vi "Dashboard Main.vi"() -> ()   [LabVIEW 2016]
uses:
  <vilib>/Utility/miscctls.llb/LVRowAndColumnTypeDef.ctl
  <vilib>/event_ctls.llb/eventvkey.ctl
  <vilib>/Rock Robotics/Network Tables/NT Read Boolean.vi
  <vilib>/Rock Robotics/WPI/Dashboard/WPI_DashboardLogging Global.vi
panel:
  in  "Camera Settings Right":T1={"Frame Rate"=30, "Compression"=30, "Size"=1, "DB Camera Config"=FALSE} {"Frame Rate" scale=1.0..30.0; "Compression" scale=100.0..-1.0; "Size" items=["640x480", "320x240", "160x120"]}
  in  "Camera Name Right":string(combo)="No Camera Selection"
  out "Camera Info":cluster{"Mbps LED":bool, "Mbps":dbl, "fps":dbl} {"fps" format="%#.1g"; "Mbps" format="%#.1g"}
  in  "Camera Settings":T1={"Frame Rate"=30, "Compression"=30, "Size"=1, "DB Camera Config"=FALSE} {"Frame Rate" scale=1.0..30.0; "Compression" scale=100.0..-1.0; "Size" items=["640x480", "320x240", "160x120"]}
  in  "TCP":refnum<k5>
  in  "Rec Mode":enum32{"Stop", "Record", "Playback"}(radio)
  out "Robot IP":string
  out "Image Message":string="Timeout in Camera Communications"
  in  "Dashboard Tab":T2(tab)
  out "?":string="CHOOSE AN AUTONOMOUS MODE!!!"
  in  "Select Auto":string(combo)="Select Autonomous ..."
  out "NT Connection":bool
  out "JS1 Z":dbl(slide) scale=-1.0..1.0 scale format="%#_2e"
  out "JS1 Graph":cluster{"X":dbl, "Y":dbl}[](graph)
  out "JS1 Buttons":T3
  out "JS2 Z":dbl(slide) scale=-1.0..1.0 scale format="%#_2e"
  out "JS2 Graph":cluster{"X":dbl, "Y":dbl}[](graph)
  out "JS2 Buttons":T3
  out "Mode":T4(ring)=enum."Auto Disabled"
  out "Camera Image Right":T5(plugin-control)
  out "Mid":dbl(slide) scale=0.0..320.0
  out "Targets Found?":bool
  out "?":string="Cortechs Robotics\nSteamworks 2017"
  out "Low Gear?":bool
  out "PID On?":bool
  out "?":dbl
  out "Time Remaining":u8(slide) scale=0.0..135.0
  out "Velocity Z":dbl(knob) scale=0.0..10.0
  out "Velocity Y":dbl(knob) scale=0.0..10.0
  out "Velocity X":dbl(knob) scale=0.0..10.0
  out "Velocity":dbl(knob) scale=0.0..10.0
  out "Acceleration Z":dbl(knob) scale=0.0..10.0
  out "Acceleration Y":dbl(knob) scale=0.0..10.0
  out "Acceleration X":dbl(knob) scale=0.0..10.0
  out "Acceleration":dbl(knob) scale=0.0..10.0
  in  "Test Slider":dbl(slide) scale=0.0..100.0 scale format="%#_3g"
  in  "On/Off":bool caption="Solenoid"
  in  "Test Name":u16(ring) items=["Select the test to run..."]
  in  "Test Tree":string(tree)
  in  "Motor":cluster{"Value":dbl, "Enable":bool} {"Value" scale=-1.0..1.0 scale format="%#_3g"}
  out "Progress":T6 {"Test Progress" scale=0.0..100.0}
  in  "Rev/Fwd":cluster{"Forward":bool, "Reverse":bool}
  in  "Test Ring":u16(ring) items=["Monochrome", "Color"]
  out "Cmd Status":string
  in  "Execute Command":bool
  in  "Command Params":string[][](table)
  in  "Command Selection":i32(listbox)
  in  "CheckList":i32(listbox)
  out "Tree":string(tree)
  out "Camera Image":T5(plugin-control)
  out "Background":bool
  in  "Camera Name":string(combo)="No Camera Selection"
  # "HW"
  # "HW"
  # "Joysticks"
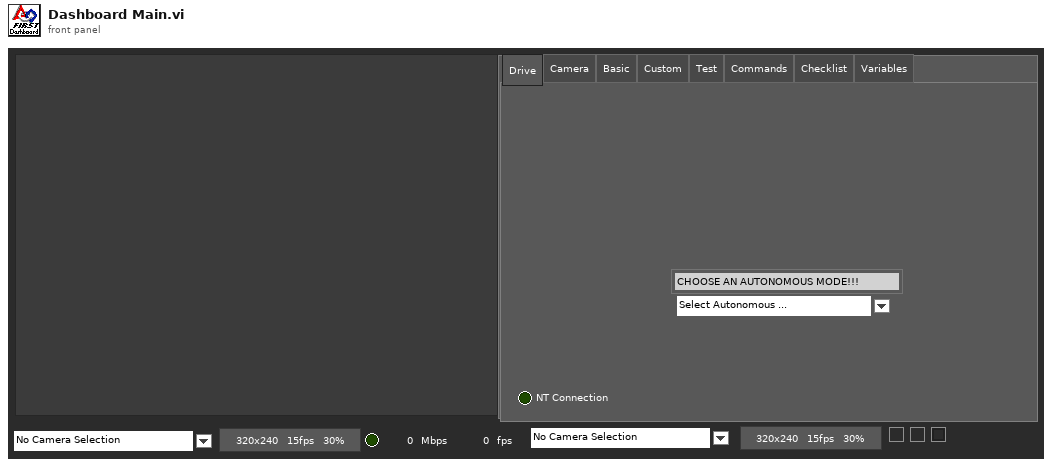
[diagram p1: front panel]
types:
  T1 = cluster{"Frame Rate":i32, "Compression":i32, "Size":u16, "DB Camera Config":bool}
  T2 = enum32{"Drive", "Camera", "Basic", "Custom", "Test", "Commands", "Checklist", "Variables"}
  T3 = cluster{bool, bool, bool, bool, bool, bool, bool, bool, bool, bool, bool, bool}
  T4 = enum8{"Tele-Op Disabled", "Tele-Op Enabled", "Auto Disabled", "Auto Enabled", "Test Disabled", "Test Enabled", "Disconnected", "No Code", "E-Stop"}
  T5 = typedef "IMAQ Image.ctl" = refnum<image>
  T6 = cluster{"Test Progress":u8, "Test Progress Text":string}
  T7 = typedef "Image Type" = u32
  T8 = cluster{"IDs":cluster{"RPC field ID":u16, "Unique ID":u16}, "String":string}
  T9 = enum32{"Drive", "Basic", "Custom", "Test", "Checklist", "Variables"}
  T10 = cluster{"Error Strings":string, "Disable Counts":cluster{u16, u16}, "Rail Faults":cluster{u16, u16, u16}, "Robot IP":string, "DB Mode":u8, "Event Info":cluster{"Name":string, "Type":u8, "Number":u16, "Replay":u8}}
  T11 = cluster{"Storage":cluster{"Disk Free":u64, "RAM Block":u32, "RAM free":u32}, "CPU Utilization":cluster{"CPU % ISR":sgl, "CPU % Time Crit":sgl, "CPU % Timed Str":sgl, "CPU % High":sgl, "CPU % Above":sgl, "CPU % Normal":sgl, "CPU % Low":sgl}, "CAN":cluster{"% Bus Utilization":sgl, "Bus Off Cnt":u32, "TX_FIFO Full Cnt":u32, "Receive Error Cnt":u8, "Transmit Error Cnt":u8}, "HID":cluster{"HID Outputs":u32, "Rumble Low":u16, "Rumble High":u16}[]}
  T12 = cluster{"Status bits":cluster{"Test Mode":bool, "Autonomous":bool, "Enabled":bool, "Code Start":bool, "Brownout":bool, "Reserved 2":bool, "Reserved 3":bool, "E-Stop":bool}, "Code Trace":cluster{"Disabled":bool, "TeleOp":bool, "Auto":bool, "Test":bool}, "Controller Type":enum16{"unknown", "cRIO", "roboRio"}, "Code?":enum16{"unknown", "noCode", "code"}, "Battery V":dbl}
  T13 = cluster{"Control Bits":cluster{"TestMode":bool, "Autonomous":bool, "Enabled":bool, "FMS Present":bool, bool, bool, bool, "E-Stop":bool}, "Team Station ":u8, "Countdown":sgl, "Joystick Values":cluster{"Axes":dbl[], "Buttons":bool[], "POVs":i16[]}[]}
  T14 = cluster{"Axes":dbl[], "Buttons":bool[], "POVs":i16[]}[]
  T15 = cluster{"Axes":dbl[], "Buttons":bool[], "POVs":i16[]}
  T16 = cluster{"Buttons[0]":bool, "Buttons[1]":bool, "Buttons[2]":bool, "Buttons[3]":bool, "Buttons[4]":bool, "Buttons[5]":bool, "Buttons[6]":bool, "Buttons[7]":bool, "Buttons[8]":bool, "Buttons[9]":bool, "Buttons[10]":bool, "Buttons[11]":bool}
  T17 = cluster{"Camera Image":refnum<vi>, "Dashboard Tab":refnum<vi>, "Background":refnum<vi>, "Rec Mode":refnum<vi>, "Test Slider":refnum<vi>, "On/Off ":refnum<vi>, "Test Ring":refnum<vi>, "Rev/Fwd":refnum<vi>, "Test Name":refnum<vi>, "Motor":refnum<vi>, "Progress":refnum<vi>, "CheckList":refnum<vi>, "Tree":refnum<vi>, "Test Tree":refnum<vi>, "Command Params":refnum<vi>, "Command Selection":refnum<vi>, "Execute Command":refnum<vi>, "Cmd Status":refnum<vi>, "Camera Settings":refnum<vi>, "Camera Name":refnum<vi>, "Camera Info":refnum<vi>, "Camera Settings Right":refnum<vi>, "Camera Name Right":refnum<vi>, "Camera Image Right":refnum<vi>}
  T18 = cluster{"Operation":enum16{"Update", "Clear"}, "Color Box":u32}[]
  T19 = typedef "eventvkey.ctl" = enum16{"ASCII", "Enter", "Return", "Shift", "Ctrl", "Alt", "Cmd", "Opt", "Caps", "NumLock", "Clear", "Break", "Up", "Down", "Left", "Right", "Insert", "Delete", "Home", "End", "PageUp", "PageDown", "Escape", "Help", "Pause", "ScrollLock", "F1", "F2", "F3", "F4", "F5", "F6", "F7", "F8", "F9", "F10", "F11", "F12", "F13", "F14", "F15", "F16", "F17", "F18", "F19", "F20", "F21", "F22", "F23", "F24", "Play", "VolumeUp", "VolumeDown", "Mute", "Two Byte Char"}
  T20 = cluster{"Image Size":bool, "Image Type":bool, "Pixel Value":bool, "ROI Information":bool, "Zoom Factor":bool}
  T21 = cluster{"Operation":enum16{"Update", "Clear"}, "Color Box":u32}
  T22 = typedef "LVRowAndColumnTypeDef.ctl" = cluster{"Row":i32, "Column":i32}
  T23 = cluster{"Shift":bool, "Ctrl":bool, "Alt":bool, "Cmd":bool, "Opt":bool}
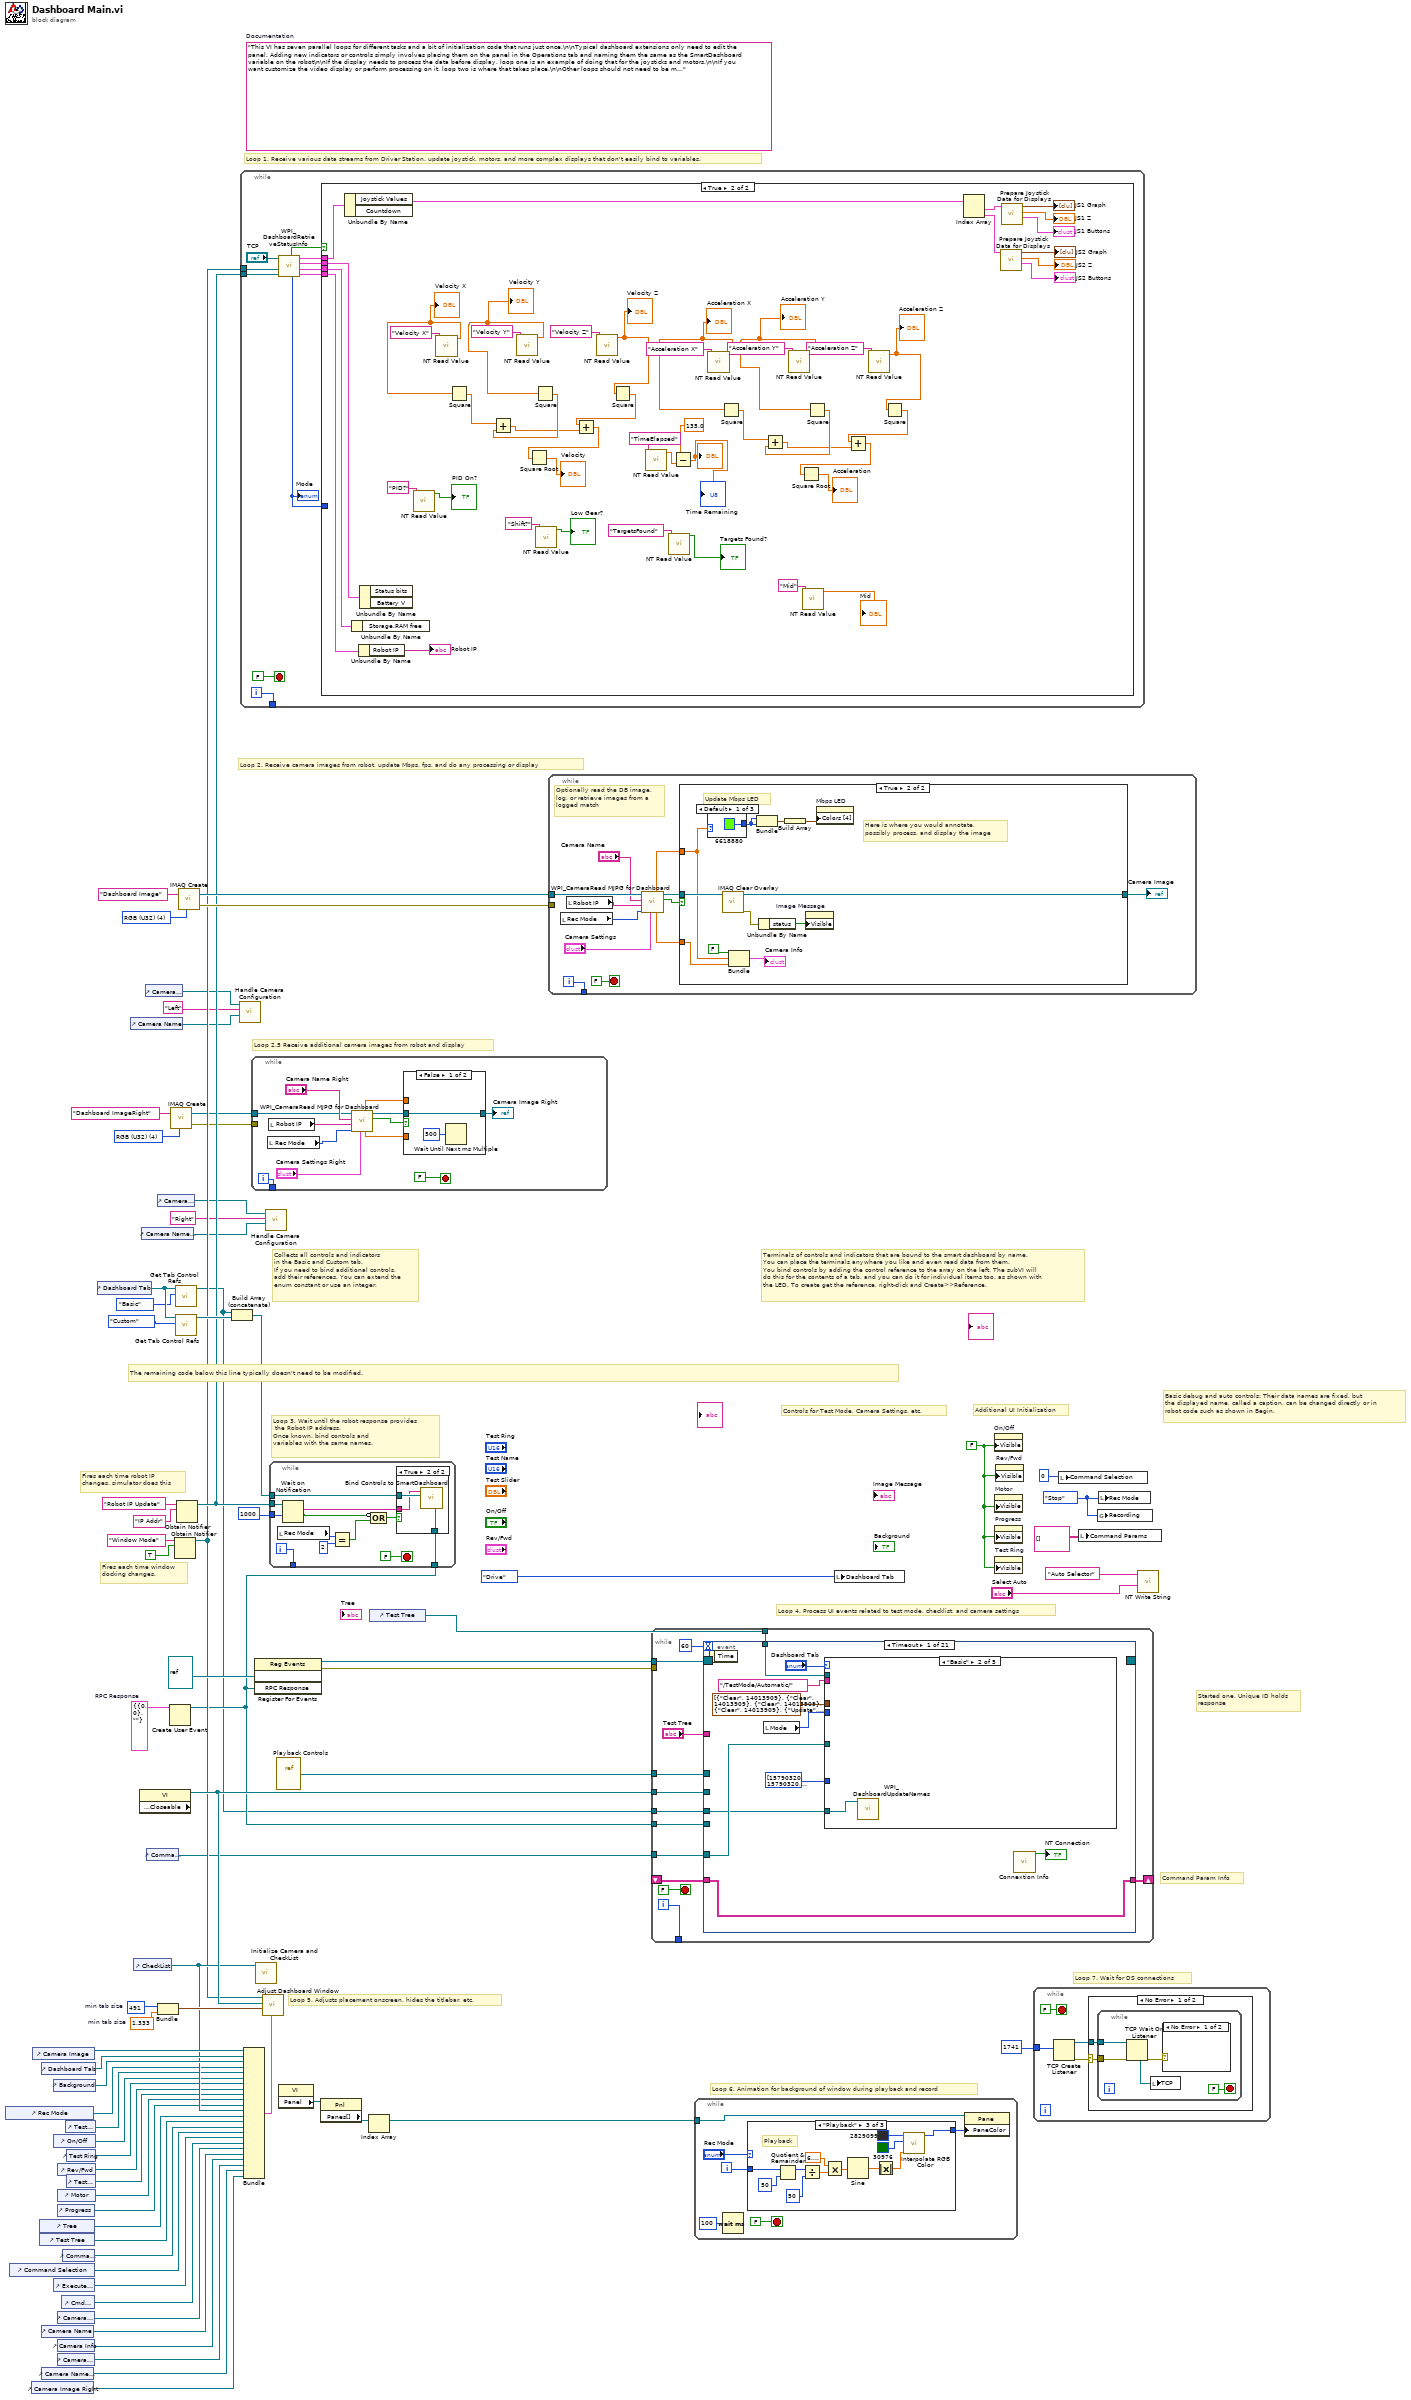
[diagram p0: block diagram]
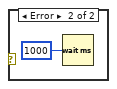
[diagram p3: hidden frame]
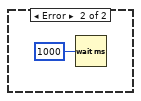
[diagram p4: hidden frame]
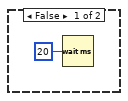
[diagram p5: hidden frame]
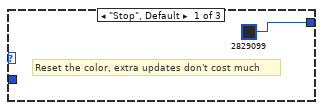
[diagram p6: hidden frame]
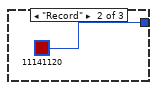
[diagram p7: hidden frame]
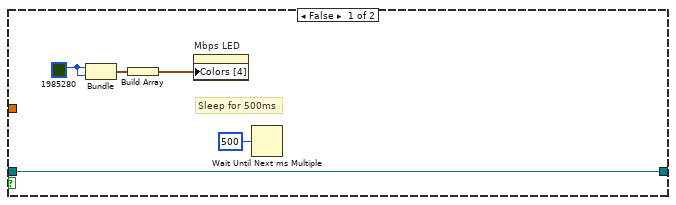
[diagram p9: hidden frame]
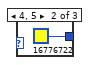
[diagram p10: hidden frame]
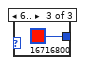
[diagram p11: hidden frame]
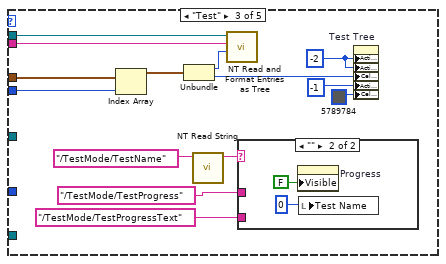
[diagram p13: hidden frame]
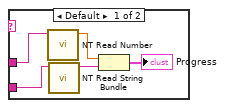
[diagram p14: hidden frame]
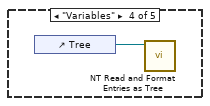
[diagram p15: hidden frame]
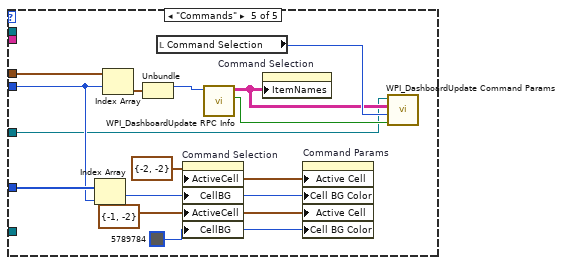
[diagram p16: hidden frame]
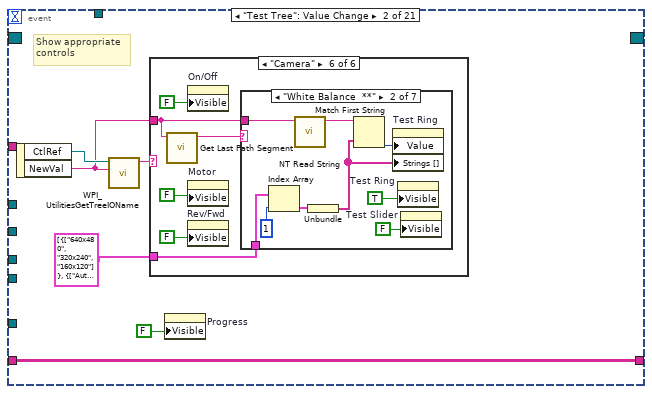
[diagram p17: hidden frame]
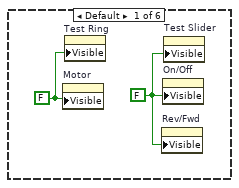
[diagram p18: hidden frame]
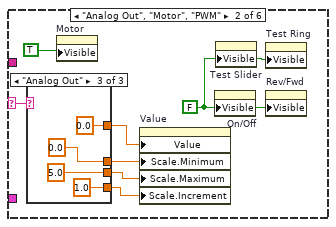
[diagram p19: hidden frame]
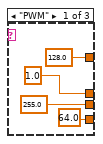
[diagram p20: hidden frame]
diagram:
  w10 = T7 4 items=["Grayscale (U8)", "Grayscale (I16)", "Grayscale (SGL)", "Complex (CSG)", "RGB (U32)", "HSL (U32)", "RGB (U64)"] ("Image Type")
  w26 = T8 {"IDs"={"RPC field ID"=0, "Unique ID"=0}, "String"=""}  # RPC Response
  w51 = 491  # min tab size
  w50 = 1.333  # min tab size
  w58 = enum32{"Stop", "Record", "Playback"}."Stop" ("Rec Mode")
  w33 = FALSE ("Visible")
  (unwired) "This VI has seven parallel loops for different tasks and a bit of initialization code that runs just once.\n\nTypical dashboard extensions only need to edit the panel. Adding new indicators or controls simply involves placing them on the panel in the Operations tab and naming them the same as the SmartDashboard variable on the robot\n\nIf the display needs to process the data before display, loop one is an example of doing that for the joysticks and motors.\n\nIf you want customize the video display or perform processing on it, loop two is where that takes place.\n\nOther loops should not need to be modified. They are pretty standard, and document the task they perform."  # Documentation
  w75 = T7 4 items=["Grayscale (U8)", "Grayscale (I16)", "Grayscale (SGL)", "Complex (CSG)", "RGB (U32)", "HSL (U32)", "RGB (U64)"] ("Image Type")
  # "Loop 2.5 Receive additional camera images from robot and display"
  # "Command Param Info"
  # "Started one, Unique ID holds\nresponse"
  # "Loop 7. Wait for DS connections"
  # "Basic debug and auto controls: Their data names are fixed, but\nthe displayed name, called a caption, can be changed directly or in\nrobot code such as shown in Begin."
  # "Controls for Test Mode, Camera Settings, etc."
  # "Additional UI Initialization"
  # "Loop 6. Animation for background of window during playback and record"
  # "Fires each time robot IP\nchanges, simulator does this"
  # "Fires each time window\ndocking changes."
  # "Collects all controls and indicators\nin the Basic and Custom tab.\nIf you need to bind additional controls,\nadd their references. You can extend the\nenum constant or use an integer."
  # "The remaining code below this line typically doesn't need to be modified."
  # "Loop 4. Process UI events related to test mode, checklist, and camera settings"
  # "Terminals of controls and indicators that are bound to the smart dashboard by name.\nYou can place the terminals anywhere you like and even read data from them.\nYou bind controls by adding the control reference to the array on the left. The subVI will\ndo this for the contents of a tab, and you can do it for individual items too, as shown with\nthe LED. To create get the reference, right-click and Create>>Reference."
  # "Loop 3. Wait until the robot response provides\n the Robot IP address.\nOnce known, bind controls and\nvariables with the same names."
  # "Loop 5. Adjusts placement onscreen, hides the titlebar, etc."
  # "Loop 1. Receive various data streams from Driver Station, update joystick, motors, and more complex displays that don't easily bind to variables."
  # "Loop 2. Receive camera images from robot, update Mbps, fps, and do any processing or display"
  n1 = control-ref of="Rec Mode"() -> (w39:refnum<vi>)
  n2 = control-ref of="Command Selection"() -> (w25:refnum<vi>)
  n3 = control-ref of="Camera Image Right"() -> (w1:refnum<vi>)
  n4 = control-ref of="Camera Image"() -> (w53:refnum<vi>)
  n5 = control-ref of="Tree"() -> (w43:refnum<vi>)
  n6 = control-ref of="Test Tree"() -> (w42:refnum<vi>)
  n7 = control-ref of="Dashboard Tab"() -> (w52:refnum<vi>)
  n8 = control-ref of="Camera Name"() -> (w16:refnum<vi>)
  n9 = control-ref of="Camera Name Right"() -> (w2:refnum<vi>)
  n10 = control-ref of="Execute Command"() -> (w27:refnum<vi>)
  n11 = control-ref of="Background"() -> (w48:refnum<vi>)
  n12 = control-ref of="On/Off"() -> (w37:refnum<vi>)
  n13 = control-ref of="Progress"() -> (w34:refnum<vi>)
  n14 = control-ref of="Camera Settings"() -> (w17:refnum<vi>)
  n15 = control-ref of="Camera Info"() -> (w15:refnum<vi>)
  n16 = control-ref of="Camera Settings Right"() -> (w3:refnum<vi>)
  n17 = control-ref of="Rev/Fwd"() -> (w35:refnum<vi>)
  n18 = control-ref of="Motor"() -> (w40:refnum<vi>)
  n19 = control-ref of="Cmd Status"() -> (w21:refnum<vi>)
  n20 = control-ref of="Command Params"() -> (w28:refnum<vi>)
  n21 = control-ref of="Test Slider"() -> (w38:refnum<vi>)
  n22 = control-ref of="Test Ring"() -> (w36:refnum<vi>)
  n23 = control-ref of="Test Name"() -> (w41:refnum<vi>)
  n24 = control-ref of="Dashboard Tab"() -> (w56:refnum<vi>)
  n25 = control-ref of="Camera Name"() -> (w18:refnum<vi>)
  n26 = control-ref of="CheckList"() -> (w44:refnum<vi>)
  n27 = property class="VI" props=["Front Panel.Closeable"]() -> (reference out=w57:refnum<vi>)  [unwired: 2 in, 2 out]
  n28 = control-ref of="Camera Name Right"() -> (w6:refnum<vi>)
  n29 = control-ref of="Camera Settings"() -> (w19:refnum<vi>)
  n30 = control-ref of="Command Params"() -> (w20:refnum<vi>)
  n31 = control-ref of="Camera Settings Right"() -> (w7:refnum<vi>)
  n32 = Bundle("min tab size"=w51, "min tab size"=w50) -> (w49:cluster{"min tab size":i32, "min tab size":dbl})  [unwired: 1 in]
  n33 = Create User Event(user event datatype=w26) -> (user event=w22:refnum<user-event>)  [unwired: 1 in, 1 out]
  n34 = call "IMAQ Create"("Image Name"="Dashboard ImageRight", "Image Type"=w10) -> ("New Image"=w9:T5, "error out"=w8:errorcluster)  [unwired: 2 in, 1 out]
  n35 = Obtain Notifier(name (unnamed)="Window Mode", notification data type=TRUE) -> (notifier out=w31:refnum<notifier>)  [unwired: 2 in, 2 out]
  n36 = call <vilib>:"Get Tab Control Refs.vi"("Page Index"=T9."Basic" ("Dashboard Tab"), "TabControl in"=w56) -> ("ControlsOnPage"=w14:refnum<vi>[])  [unwired: 9 in]
  n37 = call <vilib>:"Get Tab Control Refs.vi"("Page Index"=T9."Custom" ("Dashboard Tab"), "TabControl in"=w56) -> ("ControlsOnPage"=w55:refnum<vi>[])  [unwired: 9 in]
  n38 = Obtain Notifier(name (unnamed)="Robot IP Update", notification data type="IP Addr" ("name (unnamed)")) -> (notifier out=w32:refnum<notifier>)  [unwired: 2 in, 2 out]
  n39 = call "IMAQ Create"("Image Name"="Dashboard Image", "Image Type"=w75) -> ("New Image"=w73:T5, "error out"=w72:errorcluster)  [unwired: 2 in, 1 out]
  n40 = Build Array (concatenate)(w14, w55) -> (w54:refnum<vi>[])
  n41 = call "Handle Camera Configuration.vi"("CameraNameRef"=w18, "Camera File Name"="Left", "ClusterRef"=w19) -> ()  [unwired: 9 in]
  n42 = while {
    tunnel: [w85] -> _
    tunnel: w32 -> [w79]
    tunnel: w31 -> [w76]
    i -> [w85]
    stop <- FALSE stop-if-true
    n43 = call <vilib>:"WPI_DashboardRetrieveStatusInfo.vi"("Binding Refnum"=w79, "Window Mode Notifier"=w76, "TCP Cnx"="TCP") -> ("Power and Errors"=w80:T10, "Robot Metrics"=w83:T11, "Status Info"=w84:T12, "Control Info"=w81:T13, "Robot Mode"=w78:T4, "Process?"=w82:bool)  [unwired: 3 in]
    "Mode" <- w78
    n44 = case shown="True" w82 {
      tunnel: w84 -> [_ w137]
      tunnel: w83 -> [_ w136]
      tunnel: w81 -> [_ w135]
      tunnel: w80 -> [_ w134]
      tunnel: w78 -> [_ _]
      frame False {
        n45 = Wait (ms)(milliseconds to wait=u32 20) -> ()  [unwired: 1 out]
      }
      frame True {
        n46 = Unbundle By Name(w135) -> ("Joystick Values"=w133:T14)  [unwired: 1 out]
        n47 = Unbundle By Name(w136) -> ()  [unwired: 1 out]
        n48 = Unbundle By Name(w134) -> ("Robot IP"=→"Robot IP":string)
        n49 = Unbundle By Name(w137) -> ()  [unwired: 2 out]
        n50 = call-poly <vilib>:"NT Read Value.vi"("Name"="PID?") -> ("Boolean"=→"PID On?":bool)  [unwired: 9 in, 1 out]
        n51 = call-poly <vilib>:"NT Read Value.vi"("Name"="Velocity X") -> ("Numeric"=w114:dbl)  [unwired: 9 in, 1 out]
        "Velocity X" <- w114
        n52 = Square(x=w114) -> (x^2=w120:dbl)
        n53 = call-poly <vilib>:"NT Read Value.vi"("Name"="Velocity Y") -> ("Numeric"=w113:dbl)  [unwired: 9 in, 1 out]
        "Velocity Y" <- w113
        n54 = Square(x=w113) -> (x^2=w119:dbl)
        n55 = Add(x=w120, y=w119) -> (x+y=w118:dbl)
        n56 = call-poly <vilib>:"NT Read Value.vi"("Name"="Shift?") -> ("Boolean"=→"Low Gear?":bool)  [unwired: 9 in, 1 out]
        n57 = call-poly <vilib>:"NT Read Value.vi"("Name"="Velocity Z") -> ("Numeric"=w112:dbl)  [unwired: 9 in, 1 out]
        "Velocity Z" <- w112
        n58 = Square(x=w112) -> (x^2=w117:dbl)
        n59 = Add(x=w117, y=w118) -> (x+y=w116:dbl)
        n60 = Square Root(x=w116) -> (sqrt(x)=→"Velocity":dbl)
        n61 = call-poly <vilib>:"NT Read Value.vi"("Name"="TimeElapsed") -> ("Numeric"=w90:dbl)  [unwired: 9 in, 1 out]
        n62 = call-poly <vilib>:"NT Read Value.vi"("Name"="TargetsFound") -> ("Boolean"=→"Targets Found?":bool)  [unwired: 9 in, 1 out]
        n63 = Subtract(x=135.0, y=w90) -> (x-y=→"Time Remaining" →"?":dbl)
        n64 = call-poly <vilib>:"NT Read Value.vi"("Name"="Acceleration X") -> ("Numeric"=w102:dbl)  [unwired: 9 in, 1 out]
        "Acceleration X" <- w102
        n65 = Square(x=w102) -> (x^2=w108:dbl)
        n66 = call-poly <vilib>:"NT Read Value.vi"("Name"="Acceleration Y") -> ("Numeric"=w101:dbl)  [unwired: 9 in, 1 out]
        "Acceleration Y" <- w101
        n67 = call-poly <vilib>:"NT Read Value.vi"("Name"="Mid") -> ("Numeric"=→"Mid":dbl)  [unwired: 9 in, 1 out]
        n68 = Square(x=w101) -> (x^2=w107:dbl)
        n69 = Add(x=w108, y=w107) -> (x+y=w106:dbl)
        n70 = call-poly <vilib>:"NT Read Value.vi"("Name"="Acceleration Z") -> ("Numeric"=w100:dbl)  [unwired: 9 in, 1 out]
        "Acceleration Z" <- w100
        n71 = Square(x=w100) -> (x^2=w105:dbl)
        n72 = Add(x=w105, y=w106) -> (x+y=w104:dbl)
        n73 = Square Root(x=w104) -> (sqrt(x)=→"Acceleration":dbl)
        n74 = Index Array(array=w133) -> (element #1=w132:T15, element #2=w128:T15)  [unwired: 2 in]
        n75 = call "Prepare Joystick Data for Displays.vi"("Joystick Values"=w128) -> ("Buttons"=→"JS2 Buttons":T16, "Z Axis"=→"JS2 Z":dbl, "Cartesian Data"=→"JS2 Graph":cluster{"X axis":dbl, "X axis":dbl}[])  [unwired: 8 in]
        n76 = call "Prepare Joystick Data for Displays.vi"("Joystick Values"=w132) -> ("Buttons"=→"JS1 Buttons":T16, "Z Axis"=→"JS1 Z":dbl, "Cartesian Data"=→"JS1 Graph":cluster{"X axis":dbl, "X axis":dbl}[])  [unwired: 8 in]
      }
    }
  }
  n77 = Bundle("Camera Image"=w53, "Dashboard Tab"=w52, "Background"=w48, "Rec Mode"=w39, "Test Slider"=w38, "On/Off"=w37, "Test Ring"=w36, "Rev/Fwd"=w35, "Test Name"=w41, "Motor"=w40, "Progress"=w34, "CheckList"=w44, "Tree"=w43, "Test Tree"=w42, "Command Params"=w28, "Command Selection"=w25, "Execute Command"=w27, "Cmd Status"=w21, "Camera Settings"=w17, "Camera Name"=w16, "Camera Info"=w15, "Camera Settings Right"=w3, "Camera Name Right"=w2, "Camera Image Right"=w1) -> (w45:T17)  [unwired: 1 in]
  n78 = while {
    tunnel: w9 -> [w148]
    tunnel: w8 -> [_]
    tunnel: [w142] -> _
    i -> [w142]
    stop <- FALSE stop-if-true
    n79 = local read "Rec Mode"() -> (w146:enum32{"Stop", "Record", "Playback"})
    n80 = local read "Robot IP"() -> (w147:string)
    n81 = call <vilib>:"WPI_CameraRead MJPG for Dashboard.vi"("Camera Settings"="Camera Settings Right", "Rec Mode"=w146, "Robot IP"=w147, "Camera Name"="Camera Name Right", "Refnum in"=w148) -> ("Active"=w141:bool, "Refnum out"=w144:T5, "FPS"=w139:dbl, "Bandwidth (Mbps)"=w140:dbl)  [unwired: 3 in]
    n82 = case shown="False" w141 {
      tunnel: w144 -> [w150 w152]
      tunnel: w140 -> [_ _]
      tunnel: w139 -> [_ _]
      tunnel: [w150 w152] -> w138
      frame False {
        n83 = Wait Until Next ms Multiple(millisecond multiple=u32 500) -> ()  [unwired: 1 out]
      }
      frame True {
      }
    }
    "Camera Image Right" <- w138
  }
  n84 = register-events(refnum<vi> refnum, w22) -> (reference out=w62:refnum<event-registration>, error out=w61:errorcluster)  [unwired: 2 in]
  n85 = call "Initialize Camera and CheckList.vi"("ListBox in"=w44) -> ()  [unwired: 11 in]
  n86 = call "Adjust Dashboard Window.vi"("Sizing Refnums"=w45, "Size Constraints"=w49, "VI"=w57, "WIn Mode"=w31) -> ()  [unwired: 8 in]
  n87 = call "Handle Camera Configuration.vi"("CameraNameRef"=w6, "Camera File Name"="Right", "ClusterRef"=w7) -> ()  [unwired: 9 in]
  n88 = while {
    tunnel: w54 -> [w164]
    tunnel: w32 -> [w162]
    tunnel: [w160] -> _
    tunnel: u32 1000 ("milliseconds to wait") -> [w159]
    tunnel: w22 -> [w153]
    i -> [w160]
    stop <- FALSE stop-if-true
    n89 = local read "Rec Mode"() -> (w155:enum32{"Stop", "Record", "Playback"})
    n90 = Wait on Notification(notifier=w162, timeout in ms (-1)=w159) -> (notification=w161:string, timed out?=w157:bool)  [unwired: 2 in, 2 out]
    n91 = Equal?(x=w155, y=u16 2 ("Rec Mode")) -> (x = y?=w156:bool)
    n92 = Compound Arithmetic op=OR(invert w157, w156) -> (w158:bool)
    n93 = case shown="True" w158 {
      tunnel: w164 -> [_ w167]
      tunnel: w161 -> [_ w166]
      tunnel: w153 -> [_ w165]
      frame False {
      }
      frame True {
        n94 = call <vilib>:"Bind Controls to SmartDashboard.vi"("RPC ref"=w165, "Bound Control Refs"=w167, "Server IP Address"=w166) -> ()  [unwired: 9 in]
      }
    }
  }
  n95 = vi-ref "Playback Controls.vi"() -> (w63:refnum<vi>)
  n96 = property class="VI"() -> ("Panel"=w65:refnum<vi>)  [unwired: 2 in, 2 out]
  n97 = property class="Pnl"(reference=w65) -> ("Panes[]"=w66:refnum<vi>[])  [unwired: 1 in, 2 out]
  n98 = Index Array(array=w66) -> (element=w64:refnum<vi>)  [unwired: 1 in]
  n99 = control-ref of="Test Tree"() -> (w67:refnum<vi>)
  n100 = while {
    tunnel: w73 -> [w177]
    tunnel: w72 -> [_]
    tunnel: [w178] -> _
    i -> [w178]
    stop <- FALSE stop-if-true
    # "Optionally read the DB image,\nlog, or retrieve images from a\nlogged match"
    n101 = local read "Rec Mode"() -> (w173:enum32{"Stop", "Record", "Playback"})
    n102 = local read "Robot IP"() -> (w172:string)
    n103 = call <vilib>:"WPI_CameraRead MJPG for Dashboard.vi"("Camera Settings"="Camera Settings", "Rec Mode"=w173, "Robot IP"=w172, "Camera Name"="Camera Name", "Refnum in"=w177) -> ("Active"=w175:bool, "Refnum out"=w176:T5, "FPS"=w174:dbl, "Bandwidth (Mbps)"=w171:dbl)  [unwired: 3 in]
    n104 = case shown="True" w175 {
      tunnel: w176 -> [w180 w191]
      tunnel: w171 -> [_ w188]
      tunnel: w174 -> [_ w189]
      tunnel: [w180 w185] -> w168
      frame False {
        w182 = u32 1985280 ("Color Box")
        # "Sleep for 500ms"
        n105 = Bundle("Color Box"=w182, "Color Box"=w182) -> (w183:cluster{"Color Box":u32, "Color Box":u32})  [unwired: 1 out]
        n106 = Build Array(w183) -> (w181:cluster{"Color Box":u32, "Color Box":u32}[])
        n107 = property on="Mbps LED" class="Bool (strict)"("Colors [4]"=w181) -> ()  [unwired: 2 in, 2 out]
        n108 = Wait Until Next ms Multiple(millisecond multiple=u32 500) -> ()  [unwired: 1 out]
      }
      frame True {
        # "Here is where you would annotate,\npossibly process, and display the image"
        # "Update Mbps LED"
        n109 = case shown="Default" w188 {
          tunnel: [u32 6618880 ("Color Box") u32 16776722 ("Color Box") u32 16716800 ("Color Box")] -> w192
          frame Default {
          }
          frame 4, 5 {
          }
          frame 6.. {
          }
        }
        n110 = call "IMAQ Clear Overlay"("Image"=w191) -> ("error out"=w194:errorcluster, "Image Out"=w185:T5)  [unwired: 2 in, 7 out]
        n111 = Bundle(FALSE, "Bandwidth (Mbps)"=w188, "FPS"=w189) -> (→"Camera Info":cluster{bool, "Bandwidth (Mbps)":dbl, "FPS":dbl})  [unwired: 1 in]
        n112 = Bundle("Color Box"=w192, "Color Box"=w192) -> (w193:cluster{"Color Box":u32, "Color Box":u32})  [unwired: 1 out]
        n113 = Unbundle By Name(w194) -> ("status"=w195:bool)
        n114 = Build Array(w193) -> (w190:cluster{"Color Box":u32, "Color Box":u32}[])
        n115 = property on="Image Message" class="Str"("Visible"=w195) -> ()  [unwired: 2 in, 2 out]
        n116 = property on="Mbps LED" class="Bool (strict)"("Colors [4]"=w190) -> ()  [unwired: 2 in, 2 out]
      }
    }
    "Camera Image" <- w168
  }
  n117 = while {
    tunnel: [w208] -> _
    tunnel: w67 -> [w207]
    tunnel: w63 -> [w206]
    tunnel: w62 -> [w205]
    tunnel: w61 -> [_]
    tunnel: w57 -> [w204]
    tunnel: w22 -> [w203]
    tunnel: w20 -> [w202]
    shift-right: [w201] -> _
    shift-left: _ -> [w200]
    tunnel: w14 -> [w199]
    i -> [w208]
    stop <- FALSE stop-if-true
    n118 = event shown="[0] Timeout" {
      selector: w205 -> [_ _ _ _ _ _ _ _ _ _ _ _ _ _ _ _ _ _ _ _ _]
      dyn-events: [_ _ _ _ _ _ _ _ _ _ _ _ _ _ _ _ w464 _ _ _ _] -> _
      timeout: u32 60 ("milliseconds to wait") -> [_ _ _ _ _ _ _ _ _ _ _ _ _ _ _ _ _ _ _ _ _]
      tunnel: w207 -> [w220 _ _ _ _ _ _ _ _ _ _ _ _ _ _ _ _ _ _ _ _]
      tunnel: "Test Tree" -> [_ _ _ _ _ _ _ _ _ _ _ w431 w439 w441 w445 w453 _ _ _ _ _]
      tunnel: w206 -> [_ _ _ _ _ _ _ _ _ _ _ _ _ _ _ _ w466 _ w484 _ _]
      tunnel: w204 -> [_ _ _ _ _ _ _ _ _ _ _ _ _ _ _ _ w462 _ _ _ _]
      tunnel: w203 -> [_ _ _ _ _ _ _ _ _ _ _ _ _ _ _ _ w458 _ _ _ _]
      tunnel: w202 -> [w215 _ _ _ _ _ w382 _ _ _ _ _ _ _ _ _ _ _ _ _ _]
      tunnel: [w214 w259 w361 w366 w375 w379 w380 w389 w399 w406 w418 w430 w437 w440 w444 w452 w457 w479 w481 w485 w496] -> w201
      tunnel: w200 -> [w214 w259 w361 w366 w375 w379 w380 _ _ w406 w418 w430 w437 w440 w444 w452 w457 w479 w481 w485 w496]
      tunnel: w199 -> [w212 _ _ _ _ _ _ _ _ _ _ _ _ _ _ _ _ _ _ _ _]
      event Timeout {
        n119 = event-data() -> ()  [unwired: 1 in, 1 out]
        n120 = local read "Mode"() -> (w217:T4)
        n121 = case shown="\"Basic\"" "Dashboard Tab" {
          tunnel: w220 -> [_ _ w236 _ _]
          tunnel: "/TestMode/Automatic/" ("Name Pattern") -> [_ _ w235 _ _]
          tunnel: T18 [{"Operation"=enum."Clear", "Color Box"=14013909}, {"Operation"=enum."Clear", "Color Box"=14013909}, {"Operation"=enum."Clear", "Color Box"=14013909}, {"Operation"=enum."Clear", "Color Box"=14013909}, {"Operation"=enum."Update", "Color Box"=14013909}, {"Operation"=enum."Update", "Color Box"=16777215}, {"Operation"=enum."Clear", "Color Box"=14013909}, {"Operation"=enum."Clear", "Color Box"=14013909}, {"Operation"=enum."Clear", "Color Box"=14013909}] -> [_ _ w228 _ w252]
          tunnel: w217 -> [_ _ w227 _ w251]
          tunnel: u32[] [15790320, 15790320, 15790320, 15790320, 16777215, 16777215, 15790320, 15790320, 15790320] -> [_ _ _ _ w257]
          tunnel: w215 -> [_ _ _ _ w245]
          tunnel: w212 -> [_ w222 _ _ _]
          frame "Custom", Default {
          }
          frame "Basic" {
            n122 = call <vilib>:"WPI_DashboardUpdateNames.vi"("Controls on Tab"=w222) -> ()  [unwired: 11 in]
          }
          frame "Test" {
            w234 = -2 ("Active Item:Row Number")
            n123 = Index Array(array=w228, index=w227) -> (element=w229:T21)
            n124 = Unbundle(w229) -> ("Operation"=w230:enum16{"Update", "Clear"}, "Color Box"=w231:u32)
            n125 = call <vilib>:"NT Read String.vi"("Name"="/TestMode/TestName") -> ("String"=w225:string)  [unwired: 9 in, 1 out]
            n126 = call <vilib>:"NT Read and Format Entries as Tree.vi"("Operation"=w230, "Name Pattern"=w235, "Tree Refnum"=w236) -> ()  [unwired: 7 in, 2 out]
            n127 = case shown="\"\"" w225 {
              tunnel: "/TestMode/TestProgress" ("Name") -> [w238 _]
              tunnel: "/TestMode/TestProgressText" ("Name") -> [w237 _]
              frame Default {
                n128 = call <vilib>:"NT Read Number.vi"("Name"=w238) -> ("Numeric"=w239:dbl)  [unwired: 9 in, 1 out]
                n129 = call <vilib>:"NT Read String.vi"("Name"=w237) -> ("String"=w240:string)  [unwired: 9 in, 1 out]
                n130 = Bundle("Numeric"=w239, "String"=w240) -> (→"Progress":cluster{"Numeric":dbl, "String":string})  [unwired: 1 in]
              }
              frame "" {
                n131 = property on="Progress" class="Clust (strict)"("Visible"=FALSE) -> ()  [unwired: 2 in, 2 out]
                n132 = local write "Test Name"(u16 0) -> ()
              }
            }
            n133 = property on="Test Tree" class="Tree (strict)"("Active Item Row Number"=w234, "ActiveColNum"=w234, "CellBG"=w231, "Active Item Row Number"=-1 ("Active Item:Row Number"), "CellBG"=u32 5789784 ("Color Box")) -> ()  [unwired: 2 in, 2 out]
          }
          frame "Variables" {
            n134 = control-ref of="Tree"() -> (w244:refnum<vi>)
            n135 = call <vilib>:"NT Read and Format Entries as Tree.vi"("Tree Refnum"=w244) -> ()  [unwired: 9 in, 2 out]
          }
          frame "Commands" {
            w253 = u32 5789784 ("Color Box")
            w254 = T22 {"Row"=-1, "Column"=-2} ("Active Cell:Active Cell")
            w256 = T22 {"Row"=-2, "Column"=-2} ("Active Cell:Active Cell")
            n136 = Index Array(array=w257, index=w251) -> (element=w255:u32)
            n137 = Index Array(array=w252, index=w251) -> (element=w250:T21)
            n138 = Unbundle(w250) -> ("Operation"=w249:enum16{"Update", "Clear"})  [unwired: 1 out]
            n139 = local read "Command Selection"() -> (w248:i32)
            n140 = property on="Command Selection" class="MCListbox (strict)"("ActiveCell"=w256, "CellBG"=w255, "ActiveCell"=w254, "CellBG"=w253) -> ()  [unwired: 2 in, 2 out]
            n141 = call <vilib>:"WPI_DashboardUpdate RPC Info.vi"("Operation"=w249) -> ("update"=w247:bool, "commands"=w246:string[][])  [unwired: 9 in]
            n142 = property on="Command Selection" class="MCListbox (strict)"("ItemNames"=w246) -> ()  [unwired: 2 in, 2 out]
            n143 = property on="Command Params" class="Tbl (strict)"("Active Cell"=w256, "Cell BG Color"=w255, "Active Cell"=w254, "Cell BG Color"=w253) -> ()  [unwired: 2 in, 2 out]
            n144 = call <vilib>:"WPI_DashboardUpdate Command Params.vi"("Update"=w247, "NewVal"=w248, "Commands"=w246, "Param Tbl"=w245) -> ()  [unwired: 7 in, 1 out]
          }
        }
        n145 = call <vilib>:"Connextion Info.vi"() -> ("Connected"=→"NT Connection":bool)  [unwired: 10 in, 1 out]
      }
      event "Test Tree": Value Change {
        # "Show appropriate\ncontrols"
        n146 = event-data() -> ("CtlRef"=w262:refnum<vi>, "NewVal"=w260:string)  [unwired: 1 in]
        n147 = call <vilib>:"WPI_UtilitiesGetTreeIOName.vi"("NewVal"=w260, "TreeControl in"=w262) -> ("I/O Name"=w263:string)  [unwired: 9 in]
        n148 = case shown="\"Camera\"" w263 {
          selector: w263 -> [_ w270 _ w292 w301 _]
          tunnel: w260 -> [_ _ w289 w291 _ w308]
          tunnel: cluster{string[]}[] [{["640x480", "320x240", "160x120"]}, {["Auto", "Fixed indoor", "Fixed outdoor 1", "Fixed outdoor 2", "Fixed fluorescent 1", "Fixed fluorescent 2", "Hold current"]}, {["Auto", "Flicker-free 50 Hz", "Flicker-free 60 Hz", "Hold current"]}, {["None", "Prioritize frame rate", "Prioritize image quality"]}, {["Monochrome", "Color"]}] -> [_ _ _ _ _ w307]
          frame Default {
            w265 = FALSE ("Visible")
            w264 = FALSE ("Visible")
            n149 = property on="Motor" class="Clust (strict)"("Visible"=w264) -> ()  [unwired: 2 in, 2 out]
            n150 = property on="Test Ring" class="Ring (strict)"("Visible"=w264) -> ()  [unwired: 2 in, 2 out]
            n151 = property on="Rev/Fwd" class="Clust (strict)"("Visible"=w265) -> ()  [unwired: 2 in, 2 out]
            n152 = property on="On/Off" class="Bool (strict)"("Visible"=w265) -> ()  [unwired: 2 in, 2 out]
            n153 = property on="Test Slider" class="Slide (strict)"("Visible"=w265) -> ()  [unwired: 2 in, 2 out]
          }
          frame "Analog Out", "Motor", "PWM" {
            w271 = FALSE ("Visible")
            n154 = case shown="\"Analog Out\"" w270 {
              tunnel: [1.0 ("Value") -1.0 ("Value") 0.0 ("Value")] -> w269
              tunnel: [255.0 ("Value") 1.0 ("Value") 5.0 ("Value")] -> w268
              tunnel: [128.0 ("Value") 0.0 ("Value") 0.0 ("Value")] -> w267
              tunnel: [64.0 ("Value") 0.5 ("Value") 1.0 ("Value")] -> w266
              frame "PWM" {
              }
              frame "Motor", Default {
              }
              frame "Analog Out" {
              }
            }
            n155 = property on="Motor" class="Clust (strict)"("Visible"=TRUE) -> ()  [unwired: 2 in, 2 out]
            n156 = property on="Value" class="Slide (strict)"("Value"=w267, "Scale.Minimum"=w269, "Scale.Maximum"=w268, "Scale.Increment"=w266) -> ()  [unwired: 2 in, 2 out]
            n157 = property on="On/Off" class="Bool (strict)"("Visible"=w271) -> ()  [unwired: 2 in, 2 out]
            n158 = property on="Test Slider" class="Slide (strict)"("Visible"=w271) -> ()  [unwired: 2 in, 2 out]
            n159 = property on="Test Ring" class="Ring (strict)"("Visible"=w271) -> ()  [unwired: 2 in, 2 out]
            n160 = property on="Rev/Fwd" class="Clust (strict)"("Visible"=w271) -> ()  [unwired: 2 in, 2 out]
          }
          frame "Servo" {
            w287 = FALSE ("Visible")
            n161 = call <vilib>:"NT Read Number.vi"("Name"=w289) -> ("Numeric"=w288:dbl)  [unwired: 9 in, 1 out]
            n162 = property on="Test Slider" class="Slide (strict)"("Visible"=TRUE, "Scale.Maximum"=170.0 ("Scale.Range:Maximum")) -> ()  [unwired: 2 in, 2 out]
            n163 = local write "Test Slider"(w288) -> ()
            n164 = property on="Motor" class="Clust (strict)"("Visible"=w287) -> ()  [unwired: 2 in, 2 out]
            n165 = property on="Rev/Fwd" class="Clust (strict)"("Visible"=w287) -> ()  [unwired: 2 in, 2 out]
            n166 = property on="On/Off" class="Bool (strict)"("Visible"=w287) -> ()  [unwired: 2 in, 2 out]
            n167 = property on="Test Ring" class="Ring (strict)"("Visible"=w287) -> ()  [unwired: 2 in, 2 out]
          }
          frame "Relay", "Solenoid" {
            w290 = FALSE ("Visible")
            n168 = property on="Motor" class="Clust (strict)"("Visible"=w290) -> ()  [unwired: 2 in, 2 out]
            n169 = property on="Test Slider" class="Slide (strict)"("Visible"=w290) -> ()  [unwired: 2 in, 2 out]
            n170 = Search and Replace String(input string=w291, search string="/Value  **", replace string="/Direction") -> (result string=w297:string)  [unwired: 5 in, 3 out]
            n171 = property on="Test Ring" class="Ring (strict)"("Visible"=w290) -> ()  [unwired: 2 in, 2 out]
            n172 = call <vilib>:"NT Read String.vi"("Name"=w297) -> ("String"=w295:string)  [unwired: 9 in, 1 out]
            n173 = Equal?(x="Both directions", y=w295) -> (x = y?=w293:bool)
            n174 = Not(x=w293) -> (.not. x?=w294:bool)
            n175 = property on="Rev/Fwd" class="Clust (strict)"("Visible"=w293) -> ()  [unwired: 2 in, 2 out]
            n176 = property on="On/Off" class="Bool (strict)"("Visible"=w294, "Caption.Text"=w292) -> ()  [unwired: 2 in, 2 out]
          }
          frame "Compressor", "Digital Out" {
            w300 = FALSE ("Visible")
            # "Get direction and finish"
            n177 = property on="Motor" class="Clust (strict)"("Visible"=w300) -> ()  [unwired: 2 in, 2 out]
            n178 = property on="Test Slider" class="Slide (strict)"("Visible"=w300) -> ()  [unwired: 2 in, 2 out]
            n179 = property on="Test Ring" class="Ring (strict)"("Visible"=w300) -> ()  [unwired: 2 in, 2 out]
            n180 = property on="On/Off" class="Bool (strict)"("Visible"=TRUE, "Caption.Text"=w301) -> ()  [unwired: 2 in, 2 out]
            n181 = property on="Rev/Fwd" class="Clust (strict)"("Visible"=FALSE) -> ()  [unwired: 2 in, 2 out]
          }
          frame "Camera" {
            n182 = call <vilib>:"Get Last Path Segment.vi"("String in"=w308) -> ("String out"=w309:string)  [unwired: 10 in]
            n183 = property on="On/Off" class="Bool (strict)"("Visible"=FALSE) -> ()  [unwired: 2 in, 2 out]
            n184 = property on="Motor" class="Clust (strict)"("Visible"=FALSE) -> ()  [unwired: 2 in, 2 out]
            n185 = property on="Rev/Fwd" class="Clust (strict)"("Visible"=FALSE) -> ()  [unwired: 2 in, 2 out]
            n186 = case shown="\"White Balance  **\"" w309 {
              tunnel: w308 -> [w315 w324 w333 w342 w351 _ w357]
              tunnel: w307 -> [w313 w321 w330 w339 w348 _ _]
              frame "Size  **" {
                n187 = Index Array(array=w313) -> (element=w312:cluster{string[]})  [unwired: 1 in]
                n188 = call <vilib>:"NT Read String.vi"("Name"=w315) -> ("String"=w314:string)  [unwired: 9 in, 1 out]
                n189 = Unbundle(w312) -> (w310:string[])
                n190 = Match First String(2:w310, 3:w314) -> (0:w311:i32)  [unwired: 1 out]
                n191 = property on="Test Ring" class="Ring (strict)"("Value"=w311, "Strings []"=w310) -> ()  [unwired: 2 in, 2 out]
                n192 = property on="Test Ring" class="Ring (strict)"("Visible"=TRUE) -> ()  [unwired: 2 in, 2 out]
                n193 = property on="Test Slider" class="Slide (strict)"("Visible"=FALSE) -> ()  [unwired: 2 in, 2 out]
              }
              frame "White Balance  **" {
                n194 = Index Array(array=w321, index=1) -> (element=w322:cluster{string[]})
                n195 = call <vilib>:"NT Read String.vi"("Name"=w324) -> ("String"=w323:string)  [unwired: 9 in, 1 out]
                n196 = Unbundle(w322) -> (w319:string[])
                n197 = Match First String(2:w319, 3:w323) -> (0:w318:i32)  [unwired: 1 out]
                n198 = property on="Test Ring" class="Ring (strict)"("Value"=w318, "Strings []"=w319) -> ()  [unwired: 2 in, 2 out]
                n199 = property on="Test Ring" class="Ring (strict)"("Visible"=TRUE) -> ()  [unwired: 2 in, 2 out]
                n200 = property on="Test Slider" class="Slide (strict)"("Visible"=FALSE) -> ()  [unwired: 2 in, 2 out]
              }
              frame "Exposure  **" {
                n201 = Index Array(array=w330, index=2) -> (element=w331:cluster{string[]})
                n202 = call <vilib>:"NT Read String.vi"("Name"=w333) -> ("String"=w332:string)  [unwired: 9 in, 1 out]
                n203 = Unbundle(w331) -> (w327:string[])
                n204 = Match First String(2:w327, 3:w332) -> (0:w328:i32)  [unwired: 1 out]
                n205 = property on="Test Ring" class="Ring (strict)"("Value"=w328, "Strings []"=w327) -> ()  [unwired: 2 in, 2 out]
                n206 = property on="Test Ring" class="Ring (strict)"("Visible"=TRUE) -> ()  [unwired: 2 in, 2 out]
                n207 = property on="Test Slider" class="Slide (strict)"("Visible"=FALSE) -> ()  [unwired: 2 in, 2 out]
              }
              frame "Exposure Priority  **" {
                n208 = Index Array(array=w339, index=3) -> (element=w340:cluster{string[]})
                n209 = call <vilib>:"NT Read String.vi"("Name"=w342) -> ("String"=w341:string)  [unwired: 9 in, 1 out]
                n210 = Unbundle(w340) -> (w336:string[])
                n211 = Match First String(2:w336, 3:w341) -> (0:w337:i32)  [unwired: 1 out]
                n212 = property on="Test Ring" class="Ring (strict)"("Value"=w337, "Strings []"=w336) -> ()  [unwired: 2 in, 2 out]
                n213 = property on="Test Ring" class="Ring (strict)"("Visible"=TRUE) -> ()  [unwired: 2 in, 2 out]
                n214 = property on="Test Slider" class="Slide (strict)"("Visible"=FALSE) -> ()  [unwired: 2 in, 2 out]
              }
              frame "Color Enable  **" {
                n215 = Index Array(array=w348, index=4) -> (element=w349:cluster{string[]})
                n216 = call <vilib>:"NT Read String.vi"("Name"=w351) -> ("String"=w350:string)  [unwired: 9 in, 1 out]
                n217 = Unbundle(w349) -> (w345:string[])
                n218 = Match First String(2:w345, 3:w350) -> (0:w346:i32)  [unwired: 1 out]
                n219 = property on="Test Ring" class="Ring (strict)"("Value"=w346, "Strings []"=w345) -> ()  [unwired: 2 in, 2 out]
                n220 = property on="Test Ring" class="Ring (strict)"("Visible"=TRUE) -> ()  [unwired: 2 in, 2 out]
                n221 = property on="Test Slider" class="Slide (strict)"("Visible"=FALSE) -> ()  [unwired: 2 in, 2 out]
              }
              frame Default {
                n222 = property on="Test Ring" class="Ring (strict)"("Visible"=FALSE) -> ()  [unwired: 2 in, 2 out]
                n223 = property on="Test Slider" class="Slide (strict)"("Visible"=FALSE) -> ()  [unwired: 2 in, 2 out]
              }
              frame "Brightness  **", "Color Level  **", "Compression  **", "FPS  **", "Sharpness  **" {
                n224 = call <vilib>:"NT Read Number.vi"("Name"=w357) -> ("Numeric"=w356:dbl)  [unwired: 9 in, 1 out]
                n225 = local write "Test Slider"(w356) -> ()
                n226 = property on="Test Slider" class="Slide (strict)"("Visible"=TRUE, "Scale.Maximum"=100.0 ("Scale.Range:Maximum")) -> ()  [unwired: 2 in, 2 out]
                n227 = property on="Test Ring" class="Ring (strict)"("Visible"=FALSE) -> ()  [unwired: 2 in, 2 out]
              }
            }
          }
        }
        n228 = property on="Progress" class="Clust (strict)"("Visible"=FALSE) -> ()  [unwired: 2 in, 2 out]
      }
      event "Test Name": Mouse Enter {
        # "Populate the ring with the list of tests"
        n229 = event-data() -> ()  [unwired: 1 in, 1 out]
        n230 = call <vilib>:"NT Read String Array.vi"("Name"="/TestMode/TestList") -> ("String Array"=w365:string[])  [unwired: 9 in, 1 out]
        n231 = Build Array (concatenate)("Select the test to run...", w365) -> (w364:string[])
        n232 = property on="Test Name" class="Ring (strict)"("Strings []"=w364) -> ()  [unwired: 2 in, 2 out]
      }
      event "Test Name": Value Change {
        w367 = FALSE ("Visible")
        # "Tell the robot the test name to run"
        n233 = event-data() -> ("NewVal"=w371:u16)  [unwired: 1 in]
        n234 = property on="Test Name" class="Ring (strict)"() -> ("Strings []"=w372:string[])  [unwired: 2 in, 2 out]
        n235 = local write "Progress"(T6 {"Test Progress"=0, "Test Progress Text"=""} ("Progress")) -> ()
        n236 = Index Array(array=w372, index=w371) -> (element=w370:string)
        n237 = call <vilib>:"NT Write String.vi"("String"=w370, "Name"="/TestMode/TestName") -> ()  [unwired: 9 in, 1 out]
        n238 = property on="Progress" class="Clust (strict)"("Visible"=TRUE) -> ()  [unwired: 2 in, 2 out]
        n239 = property on="Motor" class="Clust (strict)"("Visible"=w367) -> ()  [unwired: 2 in, 2 out]
        n240 = property on="Test Slider" class="Slide (strict)"("Visible"=w367) -> ()  [unwired: 2 in, 2 out]
        n241 = property on="On/Off" class="Bool (strict)"("Visible"=w367) -> ()  [unwired: 2 in, 2 out]
        n242 = property on="Rev/Fwd" class="Clust (strict)"("Visible"=w367) -> ()  [unwired: 2 in, 2 out]
        n243 = property on="Test Ring" class="Ring (strict)"("Visible"=w367) -> ()  [unwired: 2 in, 2 out]
      }
      event "Select Auto": Mouse Enter {
        # "Populate the combo box with the list of autonomous options"
        n244 = event-data() -> ()  [unwired: 1 in, 1 out]
        n245 = call <vilib>:"NT Read String Array.vi"("Name"="Auto List") -> ("String Array"=w374:string[])  [unwired: 9 in, 1 out]
        n246 = property on="Select Auto" class="CmbBox"("Strings[]"=w374) -> ()  [unwired: 2 in, 2 out]
      }
      event "Select Auto": Value Change {
        # "User modified the Auto Selection. Write to NT variable so robot knows."
        n247 = event-data() -> ("NewVal"=w377:string)  [unwired: 1 in]
        n248 = call <vilib>:"NT Write String.vi"("String"=w377, "Name"="Auto Selector") -> ()  [unwired: 9 in, 1 out]
      }
      event "Command Selection": Value Change {
        # "Get the params and show in table"
        n249 = event-data() -> ("NewVal"=w383:i32)  [unwired: 1 in]
        n250 = property on="Command Selection" class="MCListbox (strict)"() -> ("ItemNames"=w381:string[][])  [unwired: 2 in, 2 out]
        n251 = call <vilib>:"WPI_DashboardUpdate Command Params.vi"("NewVal"=w383, "Commands"=w381, "Param Tbl"=w382) -> ()  [unwired: 8 in, 1 out]
      }
      event "Execute Command": Value Change {
        # "Started one, Unique ID holds\nresponse"
        n252 = event-data() -> ()  [unwired: 1 in, 1 out]
        n253 = property on="Command Selection" class="MCListbox (strict)"() -> ("ItemNames"=w394:string[][])  [unwired: 2 in, 2 out]
        n254 = Index Array(array=w394, index (row)="Command Selection", index (col)=0) -> (element=w392:string)
        n255 = call <vilib>:"Invoke Commands.vi"("Command Params"="Command Params", "Function Name"=w392) -> ("Params"=w388:u8, "Started"=w387:bool)  [unwired: 7 in, 1 out]
        n256 = Array Subset(array="Command Params", length (row)=w388) -> (w389:string[][])  [unwired: 3 in]
        n257 = Select(t="Executing" ("Cmd Status"), s=w387, f="" ("Cmd Status")) -> (s? t:f=→"Cmd Status":string)
      }
      event "Command Selection": Double Click {
        n258 = event-data() -> ("Row"=w402:i32)  [unwired: 1 in]
        n259 = property on="Command Selection" class="MCListbox (strict)"() -> ("ItemNames"=w405:string[][])  [unwired: 2 in, 2 out]
        n260 = local read "Command Params"() -> (w401:string[][])
        n261 = Index Array(array=w405, index (row)=w402, index (col)=0) -> (element=w403:string)
        n262 = call <vilib>:"Invoke Commands.vi"("Command Params"=w401, "Function Name"=w403) -> ("Params"=w400:u8, "Started"=w395:bool)  [unwired: 7 in, 1 out]
        n263 = Array Subset(array=w401, length (row)=w400) -> (w399:string[][])  [unwired: 3 in]
        n264 = Select(t="Executing" ("Cmd Status"), s=w395, f="" ("Cmd Status")) -> (s? t:f=w396:string)
        n265 = local write "Cmd Status"(w396) -> ()
      }
      event "CheckList": Double Click {
        # "Shift clears all"
        # "Update symbols on the listbox"
        n266 = event-data() -> ("PlatMods.Shift"=w407:bool, "Row"=w409:i32)  [unwired: 1 in]
        n267 = case shown="True" w407 {
          tunnel: w409 -> [w413 _]
          tunnel: 1 -> [w412 _]
          frame False {
            n268 = property on="CheckList" class="LstBox (strict)"() -> ("Item Symbols"=w411:i32[])  [unwired: 2 in, 2 out]
            n269 = Replace Array Subset(array=w411, new element=w412, index=w413) -> (w410:i32[])
            n270 = property on="CheckList" class="LstBox (strict)"("Item Symbols"=w410) -> ()  [unwired: 2 in, 2 out]
          }
          frame True {
            w414 = 0 ("Top Row")
            n271 = property on="CheckList" class="LstBox (strict)"() -> ("Number of Rows"=w416:u32)  [unwired: 2 in, 2 out]
            n272 = Initialize Array(0, w416) -> (w415:i32[])
            n273 = property on="CheckList" class="LstBox (strict)"("Top Row"=w414, "Value"=w414, "Item Symbols"=w415) -> ()  [unwired: 2 in, 2 out]
          }
        }
      }
      event "CheckList": Key Down {
        # "Update symbols on the listbox\nLeft and right keys check and uncheck"
        n274 = event-data() -> ("VKey"=w420:T19)  [unwired: 1 in]
        n275 = case shown="\"Left\", \"Right\"" w420 {
          selector: w420 -> [w425 _]
          tunnel: eventvkey."Left" ("VKey") -> [w423 _]
          frame "Left", "Right" {
            n276 = Equal?(x=w423, y=w425) -> (x = y?=w424:bool)
            n277 = Select(t=0, s=w424, f=1) -> (s? t:f=w426:i32)
            n278 = property on="CheckList" class="LstBox (strict)"() -> ("Item Symbols"=w429:i32[])  [unwired: 2 in, 2 out]
            n279 = Replace Array Subset(array=w429, new element=w426, index="CheckList") -> (w428:i32[])
            n280 = property on="CheckList" class="LstBox (strict)"("Item Symbols"=w428) -> ()  [unwired: 2 in, 2 out]
          }
          frame Default {
          }
        }
      }
      event "Motor.Enable": Value Change {
        # "When the test mode otor enable helper is set, update that\ntree row item's value"
        n281 = event-data() -> ("NewVal"=w435:bool)  [unwired: 1 in]
        n282 = Unbundle("Motor") -> ("Value"=w434:dbl)  [unwired: 1 out]
        n283 = Select(t=w434, s=w435, f=0.0) -> (s? t:f=w432:dbl)
        n284 = call <vilib>:"NT Write Number.vi"("Numeric"=w432, "Name"=w431) -> ()  [unwired: 9 in, 1 out]
      }
      event "Test Slider": Value Change {
        # "When the test mode slider helper is set, update that\ntree row item's value"
        n285 = event-data() -> ("NewVal"=w438:dbl)  [unwired: 1 in]
        n286 = call <vilib>:"NT Write Number.vi"("Numeric"=w438, "Name"=w439) -> ()  [unwired: 9 in, 1 out]
      }
      event "On/Off": Value Change {
        # "When the test mode on/off helper value is set, update that\ntree row item's value"
        n287 = event-data() -> ("NewVal"=w443:bool)  [unwired: 1 in]
        n288 = Boolean To (0,1)(Boolean=w443) -> (0, 1=w442:i16)
        n289 = call <vilib>:"NT Write Number.vi"("Numeric"=w442, "Name"=w441) -> ()  [unwired: 9 in, 1 out]
      }
      event "Rev/Fwd": Value Change {
        # "When the test mode helper value for relays is set, update that\ntree row item's value"
        n290 = event-data() -> ("NewVal.Forward"=w451:bool, "NewVal.Reverse"=w450:bool)  [unwired: 1 in]
        n291 = Boolean To (0,1)(Boolean=w451) -> (0, 1=w447:i16)
        n292 = Boolean To (0,1)(Boolean=w450) -> (0, 1=w449:i16)
        n293 = Negate(x=w449) -> (-x=w448:i16)
        n294 = Add(x=w447, y=w448) -> (x+y=w446:i16)
        n295 = call <vilib>:"NT Write Number.vi"("Numeric"=w446, "Name"=w445) -> ()  [unwired: 9 in, 1 out]
      }
      event "Test Ring": Value Change {
        # "When a test mode helper value is selected from the ring,\nset the tree item's variable to the string value"
        n296 = event-data() -> ("NewVal"=w455:u16)  [unwired: 1 in]
        n297 = property on="Test Ring" class="Ring (strict)"() -> ("Strings []"=w456:string[])  [unwired: 2 in, 2 out]
        n298 = Index Array(array=w456, index=w455) -> (element=w454:string)
        n299 = call <vilib>:"NT Write String.vi"("String"=w454, "Name"=w453) -> ()  [unwired: 9 in, 1 out]
      }
      event "Rec Mode": Value Change {
        # "Update globals for recording mode and path to read log from.\nClear when logging and let NetworkTables set path for vision to\nuse."
        n300 = event-data() -> ("NewVal"=w467:enum32{"Stop", "Record", "Playback"})  [unwired: 1 in]
        n301 = global write "WPI_DashboardLogging Global.vi" "Logging Filename"(path "") -> ()
        n302 = global write "WPI_DashboardLogging Global.vi" "Recording"(w467) -> ()
        n303 = case shown="\"Playback\"" w467 {
          tunnel: w466 -> [_ w469 w478]
          tunnel: [_ _ w477] -> w464
          tunnel: [_ _ w476] -> _
          tunnel: w462 -> [_ _ w474]
          tunnel: cluster{i32, i32} {-250, 170} -> [_ _ w473]
          tunnel: [_ _ T20 {"Image Size"=TRUE, "Image Type"=TRUE, "Pixel Value"=TRUE, "ROI Information"=TRUE, "Zoom Factor"=FALSE} ("Image Information Shown:All Elements")] -> w460
          tunnel: [_ _ TRUE ("Zoom Factor")] -> w459
          tunnel: w458 -> [_ _ w470]
          frame Default {
          }
          frame "Stop", "Record" {
            # "Place Window too"
            n304 = invoke class="VI" method="FP.Close"(reference=w469) -> (reference out=w468:refnum<vi>)  [unwired: 2 in, 2 out]
            n305 = invoke class="VI" method="Abort VI"(reference=w468) -> ()  [unwired: 2 in, 3 out]
          }
          frame "Playback" {
            n306 = call "Open Playback Panel.vi"("Offset"=w473, "DB VI Ref"=w474, "Playback in"=w478) -> ("Playback out"=w475:refnum<vi>)  [unwired: 8 in]
            n307 = register-events(w475, w470) -> (reference out=w477:refnum<event-registration>, error out=w476:errorcluster)  [unwired: 2 in]
          }
        }
        n308 = property on="Camera Image" class="ImageControl"("Image Information Shown"=w460, "Image Information Visible"=w459) -> ()  [unwired: 2 in, 2 out]
        n309 = call <vilib>:"WPI_DashboardNT Log FieldName Cache.vi"("Operation"=enum16{"Lookup/Add", "Index", "Clear"}."Clear") -> ()  [unwired: 8 in, 3 out]
      }
      event Panel Close {
        w480 = enum32{"Stop", "Record", "Playback"}."Stop" ("Rec Mode")
        # "Playback window has been closed, abort"
        n310 = event-data() -> ()  [unwired: 1 in, 4 out]
        n311 = local write "Rec Mode"(w480) -> ()
        n312 = global write "WPI_DashboardLogging Global.vi" "Recording"(w480) -> ()
      }
      event Panel Close {
        # "Abort playback window and ourself"
        n313 = event-data() -> ()  [unwired: 1 in, 4 out]
        n314 = invoke class="VI" method="FP.Close"(reference=w484) -> (reference out=w483:refnum<vi>)  [unwired: 2 in, 2 out]
        n315 = invoke class="VI" method="Abort VI"(reference=w483) -> (error out=w482:errorcluster)  [unwired: 2 in, 2 out]
        n316 = invoke class="VI" method="Abort VI"(error in=w482) -> ()  [unwired: 2 in, 3 out]
      }
      event User Event {
        n317 = event-data() -> ("IDs"=w491:cluster{"RPC field ID":u16, "Unique ID":u16}, "String"=w490:string)  [unwired: 1 in]
        n318 = Bundle("IDs"=w491, "String"=w490) -> (w489:T8)  [unwired: 1 in]
        n319 = call <vilib>:"Retrieve RPC Response.vi"("RPC Response"=w489) -> ("Output"=w487:string[][])  [unwired: 10 in]
        n320 = Build Array (concatenate)(w485, w487) -> (w486:string[][])
        n321 = local write "Command Params"(w486) -> ()
        n322 = local write "Cmd Status"("" ("Cmd Status")) -> ()
      }
      event "Tree": Double Click {
        n323 = event-data() -> ("PlatMods"=w495:T23, "Tag"=w494:string)  [unwired: 1 in]
        n324 = Unbundle(w495) -> ("Shift"=w493:bool)  [unwired: 4 out]
        n325 = Not(x=w493) -> (.not. x?=w492:bool)
        n326 = call <vilib>:"NT Update Persistence.vi"("Persistence"=w492, "Name"=w494) -> ()  [unwired: 9 in, 1 out]
      }
    }
  }
  n327 = while {
    tunnel: w64 -> [w498]
    i -> [w501]
    stop <- FALSE stop-if-true
    n328 = Wait (ms)(milliseconds to wait=u32 100) -> ()  [unwired: 1 out]
    n329 = case shown="\"Playback\"" "Rec Mode" {
      tunnel: w501 -> [_ _ w516]
      tunnel: [u32 2829099 ("Base Color") u32 11141120 ("Target Color") w505] -> w497
      frame "Stop", Default {
        # "Reset the color, extra updates don't cost much"
      }
      frame "Record" {
      }
      frame "Playback" {
        # "Playback"
        n330 = Quotient & Remainder(x=w516, y=u32 50 ("milliseconds to wait")) -> (x-y*floor(x/y)=w512:u32)  [unwired: 1 out]
        n331 = Divide(x=w512, y=u32 50 ("milliseconds to wait")) -> (x/y=w509:dbl)
        n332 = Multiply(x=6.283185307179586, y=w509) -> (x*y=w514:dbl)
        n333 = Sine(x=w514) -> (sin(x)=w513:dbl)
        n334 = Absolute Value(x=w513) -> (abs(x)=w506:dbl)
        n335 = call "Interpolate RGB Color.vi"("Proportion"=w506, "Target Color"=u32 30976, "Base Color"=u32 2829099) -> ("Result Color"=w505:u32)  [unwired: 8 in]
      }
    }
    n336 = property class="Pane"(reference=w498, "PaneColor"=w497) -> ()  [unwired: 1 in, 2 out]
  }
  n337 = local write "Dashboard Tab"(T2."Drive" ("Dashboard Tab")) -> ()
  n338 = property on="On/Off" class="Bool (strict)"("Visible"=w33) -> ()  [unwired: 2 in, 2 out]
  n339 = property on="Motor" class="Clust (strict)"("Visible"=w33) -> ()  [unwired: 2 in, 2 out]
  n340 = property on="Progress" class="Clust (strict)"("Visible"=w33) -> ()  [unwired: 2 in, 2 out]
  n341 = property on="Test Ring" class="Ring (strict)"("Visible"=w33) -> ()  [unwired: 2 in, 2 out]
  n342 = property on="Rev/Fwd" class="Clust (strict)"("Visible"=w33) -> ()  [unwired: 2 in, 2 out]
  n343 = while {
    tunnel: u16 1741 ("timeout ms (25000)") -> [w518]
    stop <- FALSE stop-if-true
    n344 = TCP Create Listener(10:w518) -> (0:w517:errorcluster, 3:w519:refnum<k5>)  [unwired: 4 in, 1 out]
    n345 = case shown="No Error" w517 {
      selector: w517 -> [w521 _]
      tunnel: w519 -> [w522 _]
      frame No Error {
        n346 = while {
          tunnel: w522 -> [w525]
          tunnel: w521 -> [w524]
          stop <- FALSE stop-if-true
          n347 = TCP Wait On Listener(8:w524, 11:w525) -> (0:w526:errorcluster, 4:w527:refnum<k5>)  [unwired: 2 in, 3 out]
          n348 = local write "TCP"(w527) -> ()
          n349 = case shown="No Error" w526 {
            frame No Error {
            }
            frame Error {
              n350 = Wait (ms)(milliseconds to wait=u32 1000) -> ()  [unwired: 1 out]
            }
          }
        }
      }
      frame Error {
        n351 = Wait (ms)(milliseconds to wait=u32 1000) -> ()  [unwired: 1 out]
      }
    }
  }
  n352 = local write "Command Selection"(u16 0 ("milliseconds to wait")) -> ()
  n353 = local write "Command Params"(string[][] [] ("Command Params")) -> ()
  n354 = global write "WPI_DashboardLogging Global.vi" "Recording"(w58) -> ()
  n355 = local write "Rec Mode"(w58) -> ()
  n356 = call <vilib>:"NT Write String.vi"("String"="Select Auto", "Name"="Auto Selector") -> ()  [unwired: 9 in, 1 out]
